vi "Main VI.vi"() -> ()   [LabVIEW 2014]
uses:
  Cell.lvclass
panel:
  out "Tabla de joc":picture[][](array[picture])
  in  "Flag":bool
  in  "STOP":bool
  in  "Uncover":bool
  in  "Coloana":dbl
  in  "Linie":dbl
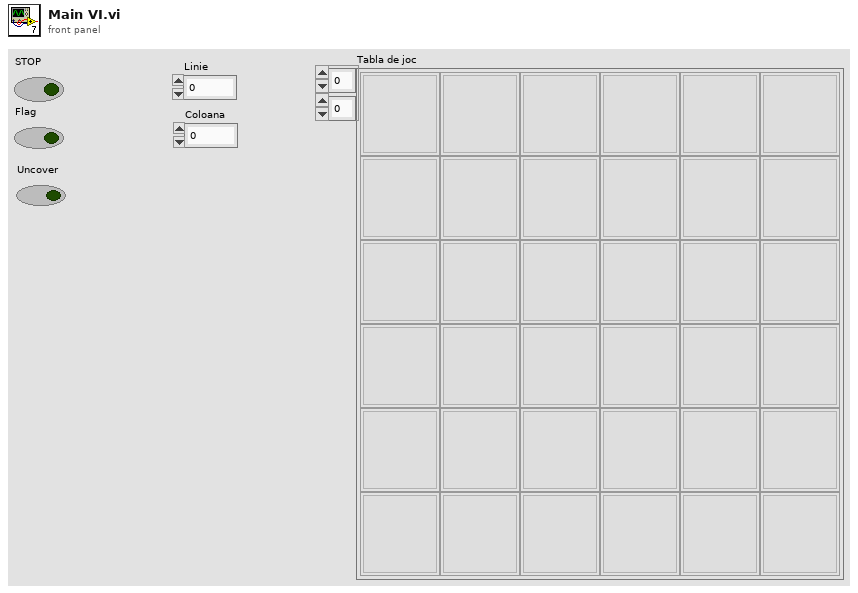
[diagram p1: front panel]
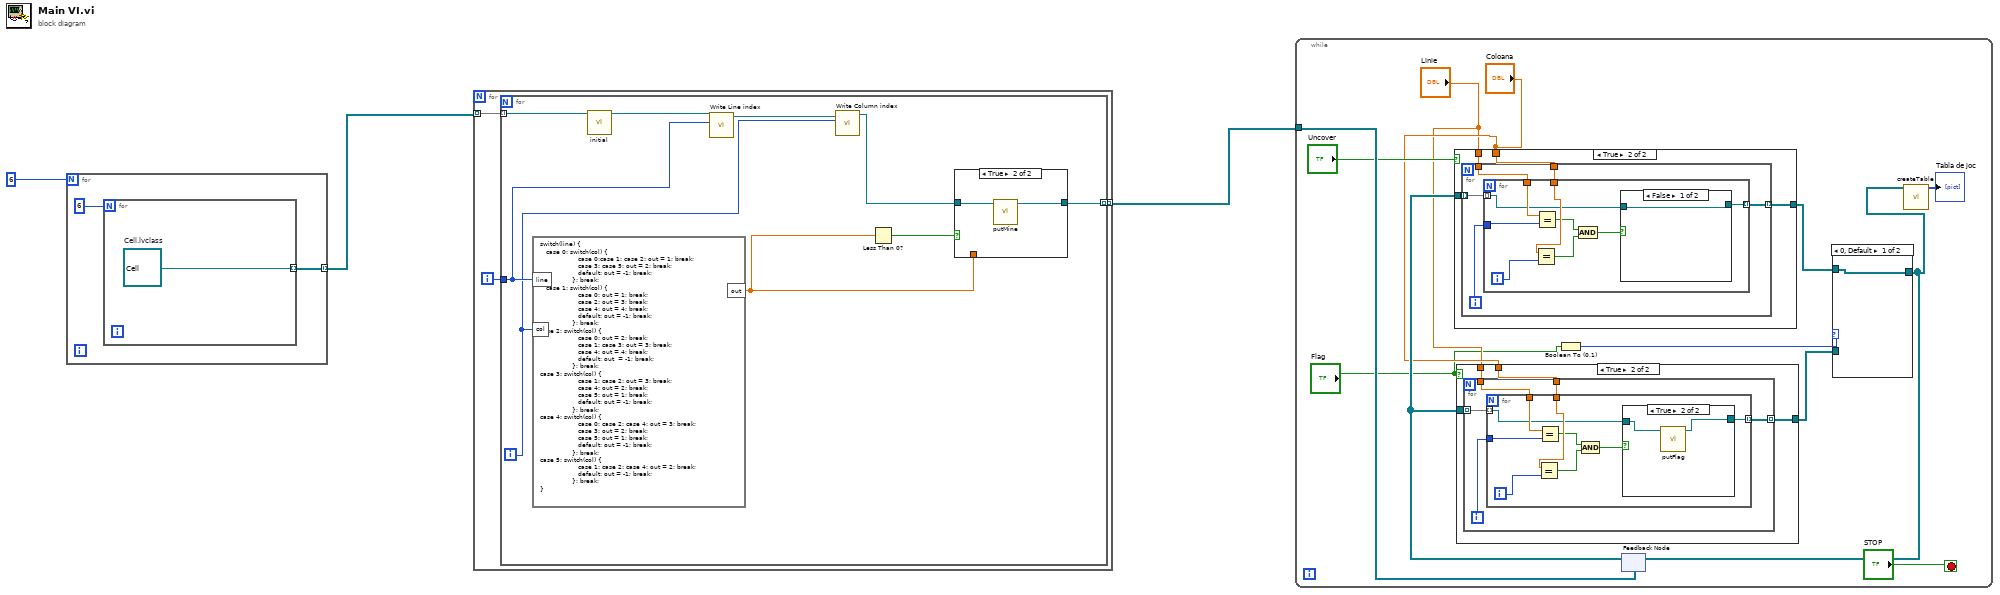
[diagram p0: block diagram]
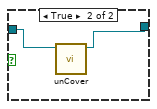
[diagram p6: hidden frame]
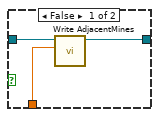
[diagram p7: hidden frame]
diagram:
  n1 = for {
    N: 6 -> [_]
    tunnel: [w4] -> w2 mode=indexing
    n2 = for {
      N: 6 -> [_]
      tunnel: [w6] -> w4 mode=indexing
      w6 = refnum<class "Cell.lvclass"> refnum  # Cell.lvclass
    }
  }
  n3 = for {
    tunnel: w2 -> [w9] mode=indexing
    tunnel: [w7] -> w1 mode=indexing
    i -> [w8]
    n4 = for {
      tunnel: w9 -> [w12] mode=indexing
      tunnel: w8 -> [w18]
      tunnel: [w10] -> w7 mode=indexing
      i -> [w16]
      n5 = formula code="switch(line) {\n   case 0: switch(col) {\n                   case 0:case 1: case 2: out = 1; break;\n                   case 3: case 5: out = 2; break;\n                   default: out = -1; break;\n                }; break;\n   case 1: switch(col) {\n                   case 0: out = 1; break;\n                   case 2: out = 3; break;\n                   case 4: out = 4; break;\n                   default: out = -1; break;\n                }; break;\ncase 2: switch(col) {\n                   case 0: out = 2; break;\n                   case 1: case 3: out = 3; break;\n                   case 4: out = 4; break;\n                   default: out  = -1; break;\n                }; break;\ncase 3: switch(col) {\n                   case 1: case 2: out = 3; break;\n                   case 4: out = 2; break;\n                   case 5: out = 1; break;\n                   default: out = -1; break;\n                }; break;\ncase 4: switch(col) {\n                   case 0: case 2: case 4: out = 3; break;\n                   case 3: out = 2; break;\n                   case 5: out = 1; break;\n                   default: out = -1; break;\n                }; break;\ncase 5: switch(col) {\n                   case 1: case 2: case 4: out = 2; break;\n                   default: out = -1; break;\n                }; break;\n}"("line"=w18, "col"=w16) -> ("out"=w14:dbl)
      n6 = call-dynamic "initial.vi"("Cell in"=w12) -> ("Cell out"=w13:refnum<class "Cell.lvclass">)  [unwired: 9 in, 1 out]
      n7 = call-dynamic "Write Line index.vi"("Line index"=w18, "Cell in"=w13) -> ("Cell out"=w17:refnum<class "Cell.lvclass">)  [unwired: 8 in, 1 out]
      n8 = call-dynamic "Write Column index.vi"("Column index"=w16, "Cell in"=w17) -> ("Cell out"=w11:refnum<class "Cell.lvclass">)  [unwired: 8 in, 1 out]
      n9 = Less Than 0?(x=w14) -> (x < 0?=w15:bool)
      n10 = case shown="True" w15 {
        tunnel: w11 -> [w21 w23]
        tunnel: [w19 w22] -> w10
        tunnel: w14 -> [w20 _]
        frame False {
          n11 = call-dynamic "Write AdjacentMines.vi"("AdjacentMines"=w20, "Cell in"=w21) -> ("Cell out"=w19:refnum<class "Cell.lvclass">)  [unwired: 8 in, 1 out]
        }
        frame True {
          n12 = call-dynamic "putMine.vi"("Cell in"=w23) -> ("Cell out"=w22:refnum<class "Cell.lvclass">)  [unwired: 9 in, 1 out]
        }
      }
    }
  }
  n13 = while {
    tunnel: w1 -> [w34]
    stop <- "STOP" stop-if-true
    n14 = Boolean To (0,1)(Boolean="Flag") -> (0, 1=w24:i16)
    n15 = feedback #1(w34) -> (w33:refnum<class "Cell.lvclass">[][])
    n16 = case shown="True" "Uncover" {
      tunnel: "Coloana" -> [_ w63]
      tunnel: "Linie" -> [_ w62]
      tunnel: w33 -> [w60 w64]
      tunnel: [w60 w61] -> w27
      frame False {
      }
      frame True {
        n17 = for {
          tunnel: w64 -> [w69] mode=indexing
          tunnel: w63 -> [w68]
          tunnel: w62 -> [w67]
          tunnel: [w65] -> w61 mode=indexing
          i -> [w66]
          n18 = for {
            tunnel: w69 -> [w71] mode=indexing
            tunnel: w68 -> [w76]
            tunnel: w67 -> [w78]
            tunnel: w66 -> [w77]
            tunnel: [w70] -> w65 mode=indexing
            i -> [w75]
            n19 = Equal?(x=w76, y=w75) -> (x = y?=w72:bool)
            n20 = Equal?(x=w78, y=w77) -> (x = y?=w73:bool)
            n21 = And(x=w73, y=w72) -> (x .and. y?=w74:bool)
            n22 = case shown="False" w74 {
              tunnel: w71 -> [w79 w81]
              tunnel: [w79 w80] -> w70
              frame False {
              }
              frame True {
                n23 = call-dynamic "unCover.vi"("Cell in"=w81) -> ("Cell out"=w80:refnum<class "Cell.lvclass">)  [unwired: 8 in, 2 out]
              }
            }
          }
        }
      }
    }
    n24 = case shown="True" "Flag" {
      tunnel: "Coloana" -> [_ w41]
      tunnel: "Linie" -> [_ w40]
      tunnel: w33 -> [w38 w42]
      tunnel: [w38 w39] -> w28
      frame False {
      }
      frame True {
        n25 = for {
          tunnel: w42 -> [w47] mode=indexing
          tunnel: w41 -> [w46]
          tunnel: w40 -> [w45]
          tunnel: [w43] -> w39 mode=indexing
          i -> [w44]
          n26 = for {
            tunnel: w47 -> [w49] mode=indexing
            tunnel: w46 -> [w54]
            tunnel: w45 -> [w56]
            tunnel: w44 -> [w55]
            tunnel: [w48] -> w43 mode=indexing
            i -> [w53]
            n27 = Equal?(x=w54, y=w53) -> (x = y?=w50:bool)
            n28 = Equal?(x=w56, y=w55) -> (x = y?=w51:bool)
            n29 = And(x=w51, y=w50) -> (x .and. y?=w52:bool)
            n30 = case shown="True" w52 {
              tunnel: w49 -> [w57 w59]
              tunnel: [w57 w58] -> w48
              frame False {
              }
              frame True {
                n31 = call-dynamic "putFlag.vi"("Cell in"=w59) -> ("Cell out"=w58:refnum<class "Cell.lvclass">)  [unwired: 9 in, 1 out]
              }
            }
          }
        }
      }
    }
    n32 = case shown="0, Default" w24 {
      tunnel: w28 -> [_ w37]
      tunnel: w27 -> [w36 _]
      tunnel: [w36 w37] -> w26
      frame 0, Default {
      }
      frame 1 {
      }
    }
    n33 = feedback-in #1(w26) -> ()
    n34 = call "createTable.vi"("Input board"=w26) -> ("Array"=→"Tabla de joc":picture[][])  [unwired: 9 in, 1 out]
  }
